vi "Configuration parameter writing.vi"(4 "Calibration angle":sgl, 6 "电子罗盘":T1={"VISA resource name"="", "baud rate (9600)"=9600, "串口打开"=FALSE} {"baud rate (9600)" items=["1200"=1200, "2400"=2400, "4800"=4800, "9600"=9600, "38400"=38400, "115200"=115200]}, 7 "Shift distance":u32, 8 "error in (no error)":errorcluster caption="错误输入（无错误）", 9 "enable":bool, 10 "baud rate (9600)":u32(ring)=4800 caption="波特率" items=["1200"=1200, "2400"=2400, "4800"=4800, "9600"=9600, "19200"=19200, "38400"=38400, "115200"=115200], 11 "VISA resource name":refnum<visa-resource-name> caption="串口") -> (0 "error out":errorcluster caption="错误输出")   [LabVIEW 2016, in "AIRMAR WeatherCaster.lvlib"]
uses:
  AIRMAR WeatherCaster.lvlib
  <vilib>/Utility/config.llb/Write Key (String).vi
  <vilib>/Utility/config.llb/Write Key (U32).vi
  <vilib>/Utility/config.llb/Write Key (Boolean).vi
  <vilib>/Utility/config.llb/Write Key (Double).vi
  <vilib>/Utility/config.llb/NI_LVConfig.lvlib
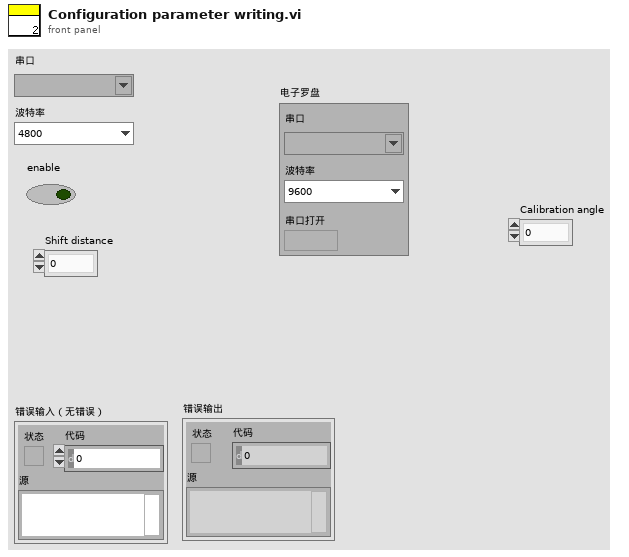
[diagram p1: front panel]
types:
  T1 = cluster{"VISA resource name":refnum<visa-resource-name>, "baud rate (9600)":u32, "串口打开":bool}
  T2 = typedef "NI_LVConfig.lvlib/Config Data RefNum.ctl" = refnum<k1>
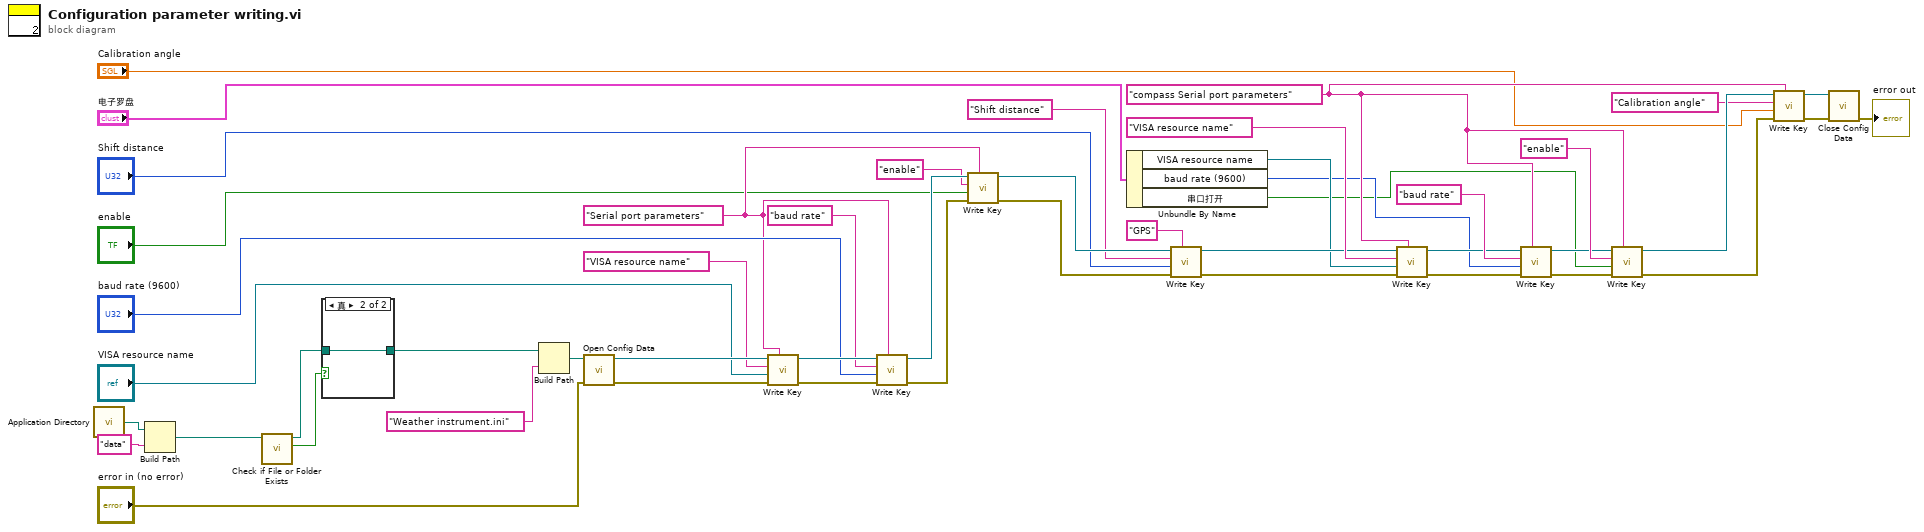
[diagram p0: block diagram]
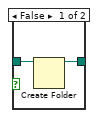
[diagram p2: hidden frame]
diagram:
  w12 = "compass Serial port parameters" ("section")
  w28 = "Serial port parameters" ("section")
  n1 = call <vilib>:"Application Directory.vi"() -> ("Application Directory"=w36:path)
  n2 = Build Path(base path=w36, name or relative path="data" ("名称或相对路径")) -> (appended path=w34:path)
  n3 = call <vilib>:"Check if File or Folder Exists.vi"("path"=w34) -> ("file or folder exists?"=w33:bool, "dup path"=w32:path)  [unwired: 8 in, 1 out]
  n4 = case shown="真" w33 {
    tunnel: w32 -> [w50 w51]
    tunnel: [w49 w51] -> w31
    frame False {
      n5 = Create Folder(path (use dialog)=w50) -> (created path=w49:path)  [unwired: 2 in, 2 out]
    }
    frame True {
    }
  }
  n6 = Build Path(base path=w31, name or relative path="Weather instrument.ini" ("名称或相对路径")) -> (appended path=w46:path)
  n7 = call <vilib>:"Open Config Data.vi"("error in (no error)"="error in (no error)", "configuration file path"=w46) -> ("error out"=w47:errorcluster, "refnum"=w48:T2)  [unwired: 7 in, 1 out]
  n8 = call-poly <vilib>:"Write Key.vi"("section"=w28, "error in (no error)"=w47, "value"="VISA resource name", "key"="VISA resource name", "refnum"=w48) -> ("error out"=w42:errorcluster, "refnum out"=w43:T2)  [unwired: 4 in, 1 out]
  n9 = call-poly <vilib>:"Write Key.vi"("section"=w28, "error in (no error)"=w42, "value"="baud rate (9600)", "key"="baud rate", "refnum"=w43) -> ("error out"=w30:errorcluster, "refnum out"=w29:T2)  [unwired: 4 in, 1 out]
  n10 = call-poly <vilib>:"Write Key.vi"("section"=w28, "error in (no error)"=w30, "value"="enable", "key"="enable", "refnum"=w29) -> ("error out"=w24:errorcluster, "refnum out"=w25:T2)  [unwired: 4 in, 1 out]
  n11 = Unbundle By Name("电子罗盘") -> ("VISA resource name"=w3:refnum<visa-resource-name>, "baud rate (9600)"=w2:u32, "串口打开"=w1:bool)
  n12 = call-poly <vilib>:"Write Key.vi"("section"="GPS", "error in (no error)"=w24, "value"="Shift distance", "key"="Shift distance" ("section"), "refnum"=w25) -> ("error out"=w7:errorcluster, "refnum out"=w8:T2)  [unwired: 4 in, 1 out]
  n13 = call-poly <vilib>:"Write Key.vi"("section"=w12, "error in (no error)"=w7, "value"=w3, "key"="VISA resource name", "refnum"=w8) -> ("error out"=w16:errorcluster, "refnum out"=w15:T2)  [unwired: 4 in, 1 out]
  n14 = call-poly <vilib>:"Write Key.vi"("section"=w12, "error in (no error)"=w16, "value"=w2, "key"="baud rate", "refnum"=w15) -> ("error out"=w18:errorcluster, "refnum out"=w19:T2)  [unwired: 4 in, 1 out]
  n15 = call-poly <vilib>:"Write Key.vi"("section"=w12, "error in (no error)"=w18, "value"=w1, "key"="enable", "refnum"=w19) -> ("error out"=w10:errorcluster, "refnum out"=w13:T2)  [unwired: 4 in, 1 out]
  n16 = call-poly <vilib>:"Write Key.vi"("section"=w12, "error in (no error)"=w10, "value"="Calibration angle", "key"="Calibration angle", "refnum"=w13) -> ("error out"=w5:errorcluster, "refnum out"=w6:T2)  [unwired: 4 in, 1 out]
  n17 = call <vilib>:"Close Config Data.vi"("error in (no error)"=w5, "refnum"=w6) -> ("error out"=→"error out":errorcluster)  [unwired: 8 in, 1 out]
